vi "SaveData Loop (numpy).vi"(8 "error in":errorcluster, 10 "Message Queues out":T13, 11 "Notifiers":T1) -> (0 "error out":errorcluster)   [LabVIEW 2014]
uses:
  support/Message Queue/All Message Queues.ctl
  support/Message Queue/Message Cluster.ctl
  support/Notifiers/Notifiers.ctl
  controls/IBM OptoElectroMechanics Message Handler Loop Notifiers.ctl
  Hardware Control/HP4155C/HP4155C Notifiers.ctl
  Hardware Control/Keithley707A/Keithley 707A Notifiers.ctl
  Hardware Control/Newport ESP301/StressControl Notifiers.ctl
  Hardware Control/NGSLabspec/LabramHR Notifiers.ctl
  Hardware Control/Switches and Mirrors/SwitchesMirrors Notifiers.ctl
  Hardware Control/Camera/Camera Notifiers.ctl
  Hardware Control/Tango XYZ Stage/Tango Notifications.ctl
  Hardware Control/Autofocus/Autofocus Notifiers.ctl
  Measurements/Save Data/SaveData Notifiers.ctl
  Measurements/Instrument Sequence/Instrument Sequence Notifiers.ctl
  Measurements/Save Data/SaveData Function.ctl
  support/Message Queue/IBM OptoElectroMechanics Message Queue.lvlib
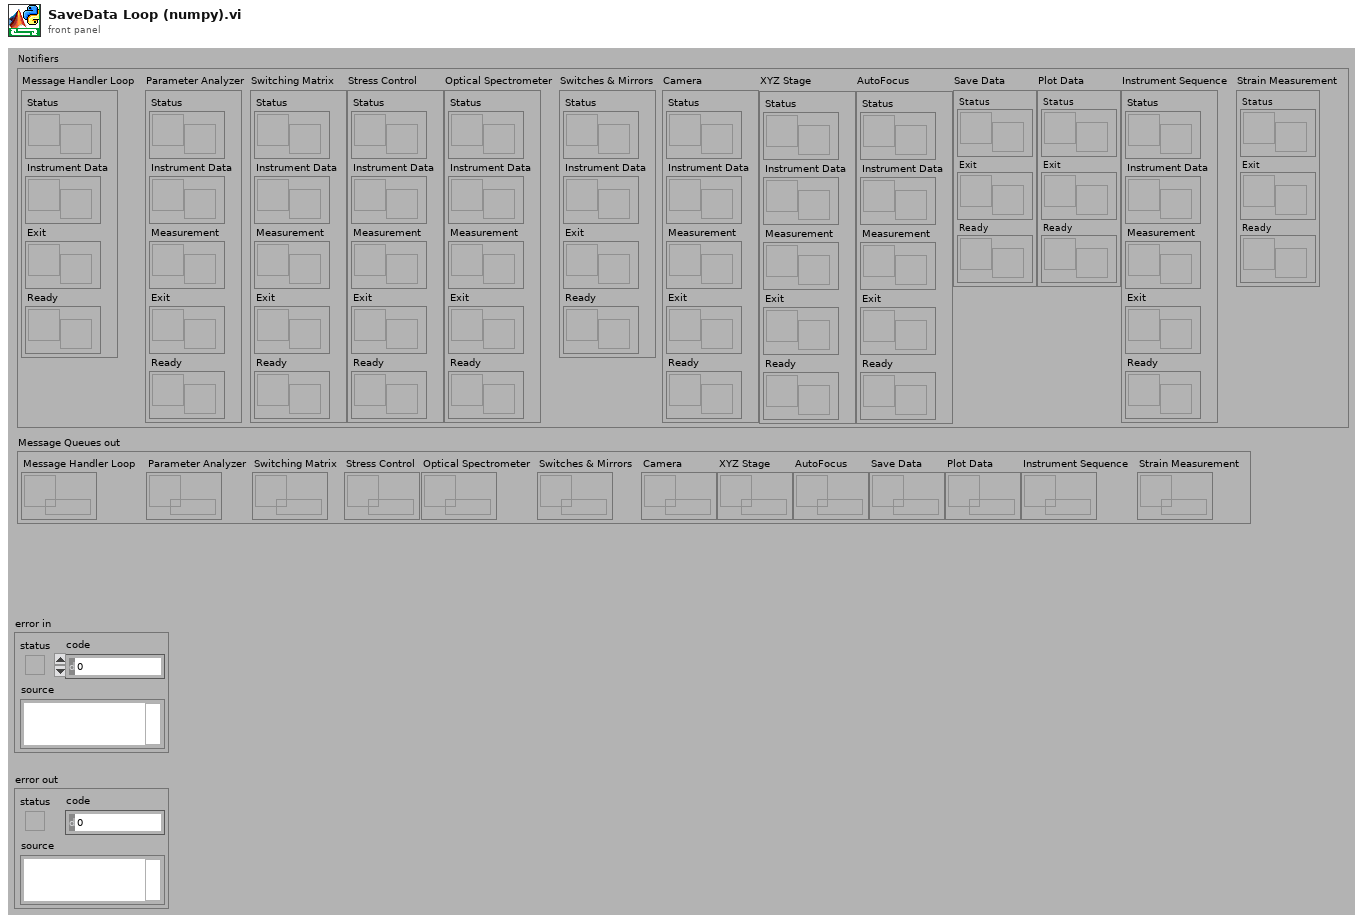
[diagram p1: front panel]
types:
  T1 = typedef "Notifiers.ctl" = cluster{"Message Handler Loop":T2, "Parameter Analyzer":T3, "Switching Matrix":T4, "Stress Control":T5, "Optical Spectrometer":T6, "Switches & Mirrors":T7, "Camera":T8, "XYZ Stage":T9, "AutoFocus":T10, "Save Data":T11, "Plot Data":T11, "Instrument Sequence":T12, "Strain Measurement":cluster{"Status":refnum<notifier>, "Exit":refnum<notifier>, "Ready":refnum<notifier>}}
  T2 = typedef "IBM OptoElectroMechanics Message Handler Loop Notifiers.ctl" = cluster{"Status":refnum<notifier>, "Instrument Data":refnum<notifier>, "Exit":refnum<notifier>, "Ready":refnum<notifier>}
  T3 = typedef "HP4155C Notifiers.ctl" = cluster{"Status":refnum<notifier>, "Instrument Data":refnum<notifier>, "Measurement":refnum<notifier>, "Exit":refnum<notifier>, "Ready":refnum<notifier>}
  T4 = typedef "Keithley 707A Notifiers.ctl" = cluster{"Status":refnum<notifier>, "Instrument Data":refnum<notifier>, "Measurement":refnum<notifier>, "Exit":refnum<notifier>, "Ready":refnum<notifier>}
  T5 = typedef "StressControl Notifiers.ctl" = cluster{"Status":refnum<notifier>, "Instrument Data":refnum<notifier>, "Measurement":refnum<notifier>, "Exit":refnum<notifier>, "Ready":refnum<notifier>}
  T6 = typedef "LabramHR Notifiers.ctl" = cluster{"Status":refnum<notifier>, "Instrument Data":refnum<notifier>, "Measurement":refnum<notifier>, "Exit":refnum<notifier>, "Ready":refnum<notifier>}
  T7 = typedef "SwitchesMirrors Notifiers.ctl" = cluster{"Status":refnum<notifier>, "Instrument Data":refnum<notifier>, "Exit":refnum<notifier>, "Ready":refnum<notifier>}
  T8 = typedef "Camera Notifiers.ctl" = cluster{"Status":refnum<notifier>, "Instrument Data":refnum<notifier>, "Measurement":refnum<notifier>, "Exit":refnum<notifier>, "Ready":refnum<notifier>}
  T9 = typedef "Tango Notifications.ctl" = cluster{"Status":refnum<notifier>, "Instrument Data":refnum<notifier>, "Measurement":refnum<notifier>, "Exit":refnum<notifier>, "Ready":refnum<notifier>}
  T10 = typedef "Autofocus Notifiers.ctl" = cluster{"Status":refnum<notifier>, "Instrument Data":refnum<notifier>, "Measurement":refnum<notifier>, "Exit":refnum<notifier>, "Ready":refnum<notifier>}
  T11 = typedef "SaveData Notifiers.ctl" = cluster{"Status":refnum<notifier>, "Exit":refnum<notifier>, "Ready":refnum<notifier>}
  T12 = typedef "Instrument Sequence Notifiers.ctl" = cluster{"Status":refnum<notifier>, "Instrument Data":refnum<notifier>, "Measurement":refnum<notifier>, "Exit":refnum<notifier>, "Ready":refnum<notifier>}
  T13 = typedef "IBM OptoElectroMechanics Message Queue.lvlib/All Message Queues.ctl" = cluster{"Message Handler Loop":refnum<queue>, "Parameter Analyzer":refnum<queue>, "Switching Matrix":refnum<queue>, "Stress Control":refnum<queue>, "Optical Spectrometer":refnum<queue>, "Switches & Mirrors":refnum<queue>, "Camera":refnum<queue>, "XYZ Stage":refnum<queue>, "AutoFocus":refnum<queue>, "Save Data":refnum<queue>, "Plot Data":refnum<queue>, "Instrument Sequence":refnum<queue>, "Strain Measurement":refnum<queue>}
  T14 = typedef "SaveData Function.ctl" = enum16{"Start Python Session", "Set Data Structures to Default", "Append Stress Data", "Append Electrical Measurement", "Append Optical Spectrum", "Append Stress Measurement Step", "Append Instrument Sequence Step", "Set Instrument Configuration", "Set Stress Data", "Set Electrical Measurement", "Set Optical Spectum", "Save Electrical Measurement", "Save Optical Spectrum", "Save Instrument Sequence", "Save Stress Measurement", "Pickle2Workspace", "Explore Variable Space", "Close"}
  T15 = typedef "SaveData Data.ctl" = cluster{"Configuration":T16, "Initialization":T21}
  T16 = typedef "SaveData Config.ctl" = cluster{"Workspace Info":T17, "Instrument Configuration":T18, "Stress Motor Position":dbl, "Electrical Measurement":cluster{"Sequence":dbl[], "V1":dbl[], "V2":dbl[], "V3":dbl[], "V4":dbl[], "I1":dbl[], "I2":dbl[], "I3":dbl[], "I4":dbl[]}, "Optical Spectrum":T20}
  T17 = typedef "SaveData Workspace Info.ctl" = cluster{"Device Name":string, "Device Info":string, "Path":path}
  T18 = typedef "SaveData Instrument Configuration.ctl" = cluster{"Instrument":T19, "Configuration":string}
  T19 = typedef "Instrument List.ctl" = enum32{"Unknown Instrument", "Switching Matrix", "Parameter Analyzer", "Optical Spectrometer"}
  T20 = typedef "Spectral Data.ctl" = cluster{"Intensity":dbl[], "Wavelength":dbl[], "Energy":dbl[], "Raman Shift":dbl[], "Detector Temperature":dbl}
  T21 = typedef "SaveData Initialization.ctl" = cluster{"Start Python Session":bool, "Set Datastructures to Default":bool}
  T22 = cluster{"Sequence":dbl[], "V1":dbl[], "V2":dbl[], "V3":dbl[], "V4":dbl[], "I1":dbl[], "I2":dbl[], "I3":dbl[], "I4":dbl[]}
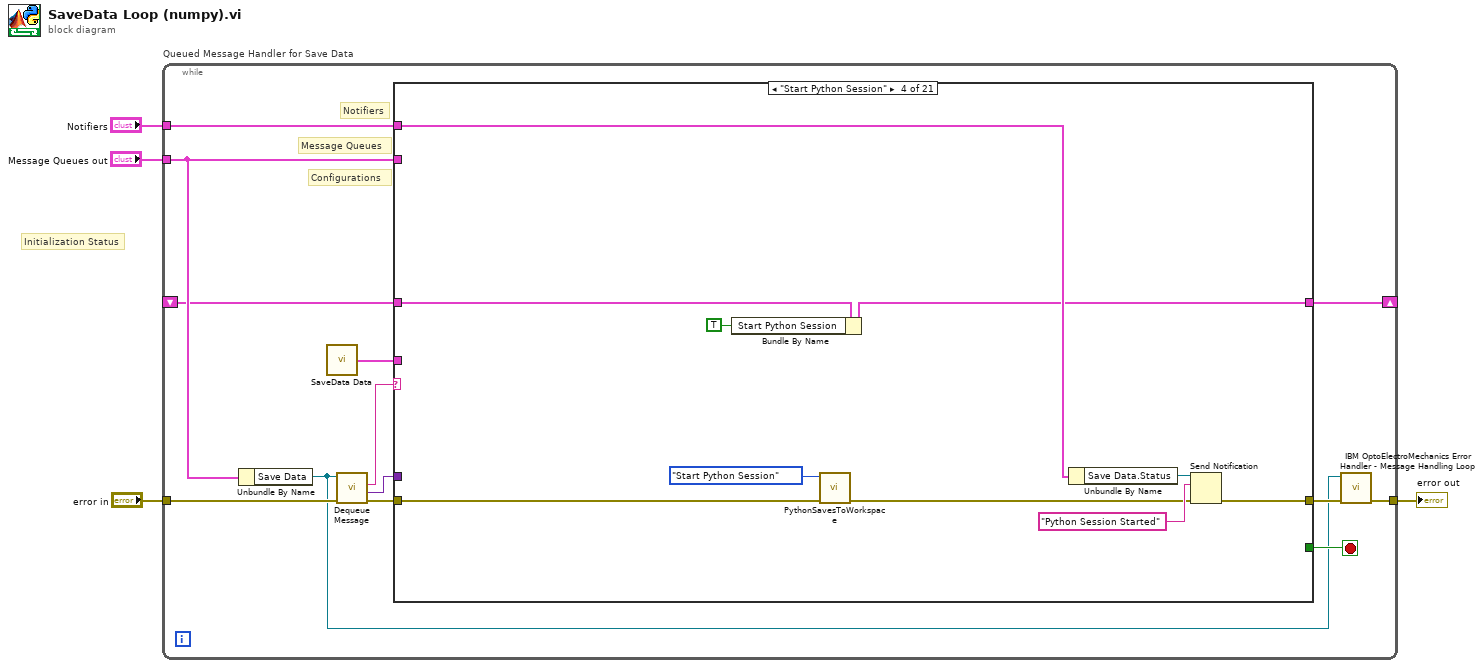
[diagram p0: block diagram]
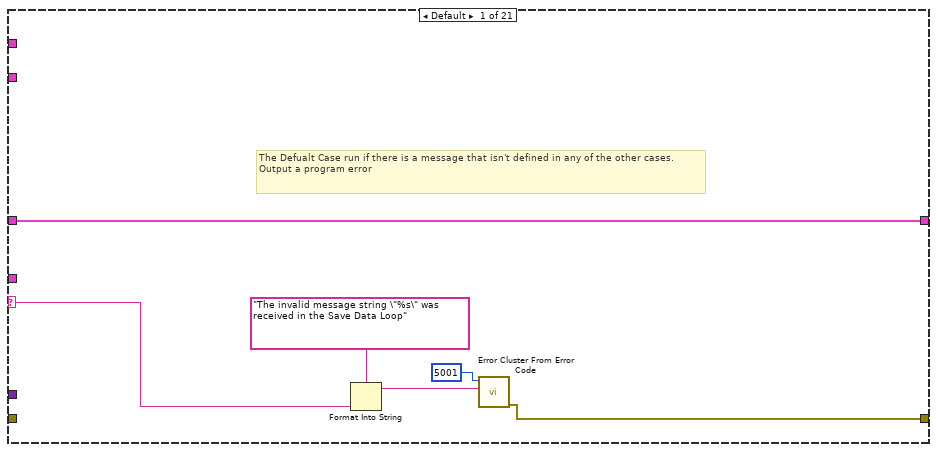
[diagram p2: hidden frame]
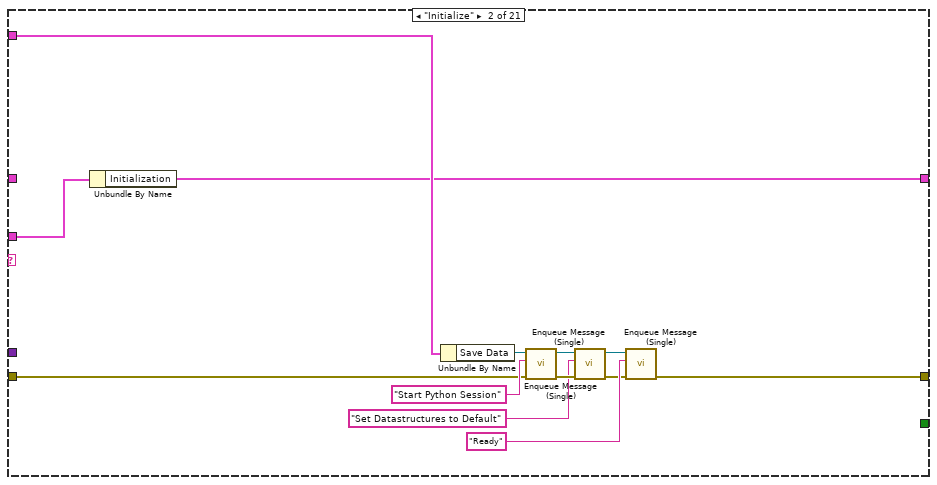
[diagram p3: hidden frame]
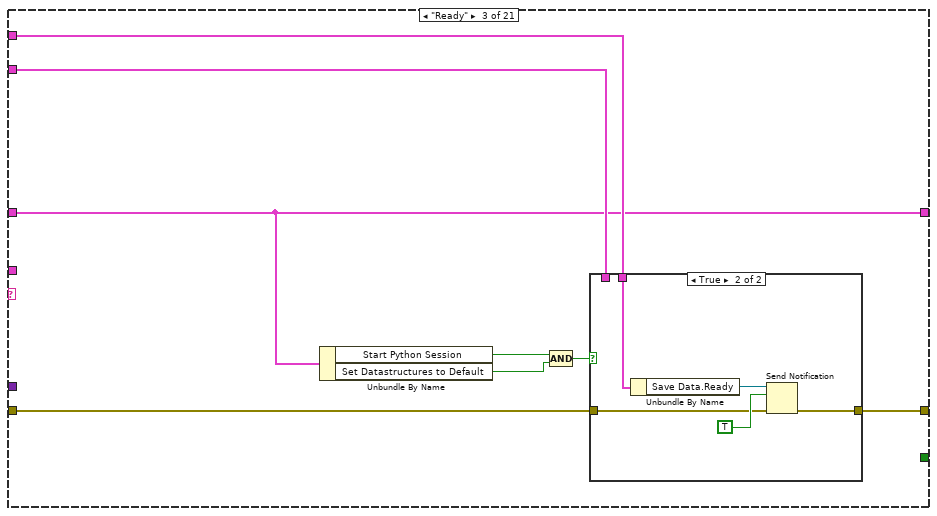
[diagram p4: hidden frame]
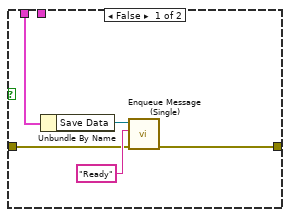
[diagram p5: hidden frame]
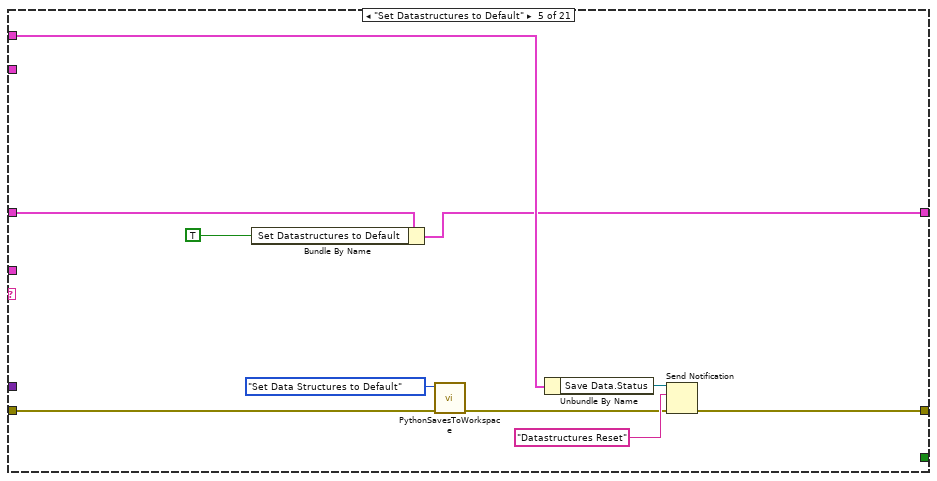
[diagram p6: hidden frame]
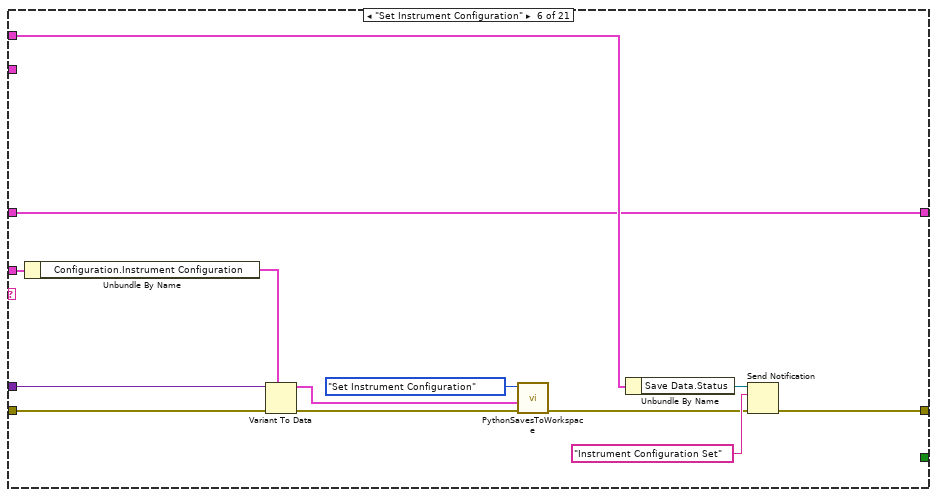
[diagram p7: hidden frame]
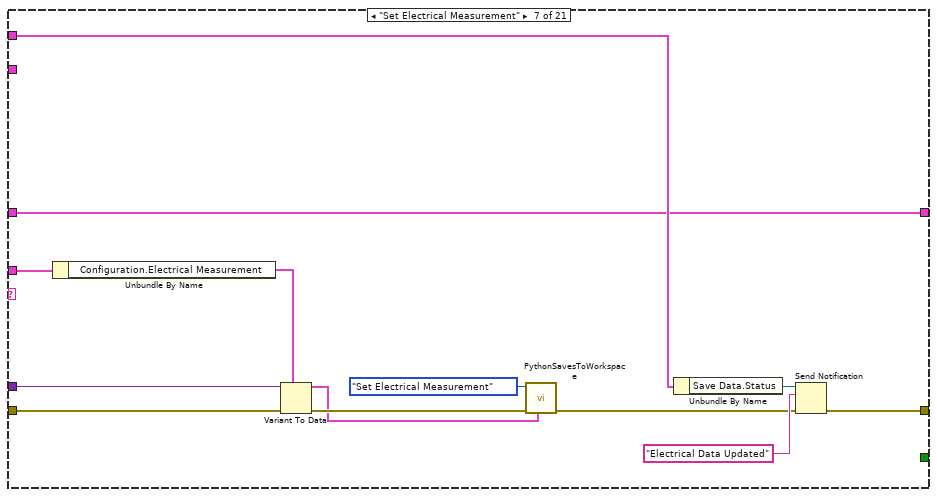
[diagram p8: hidden frame]
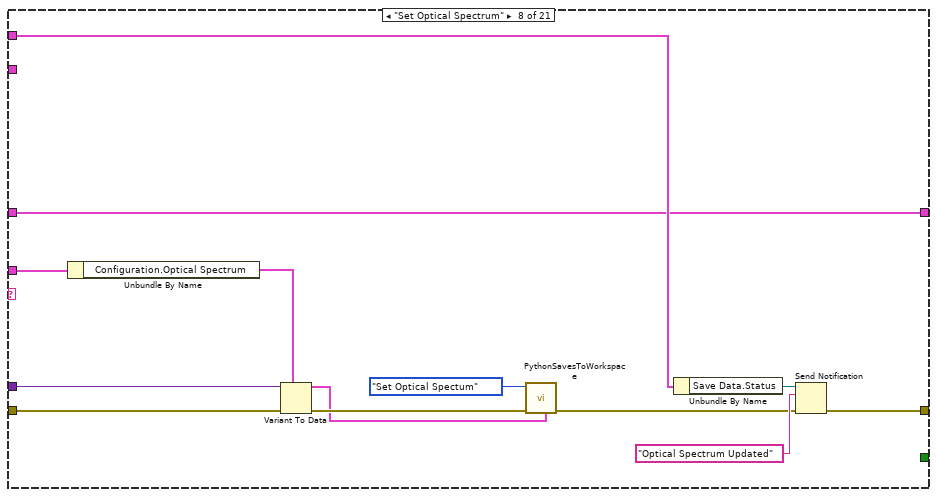
[diagram p9: hidden frame]
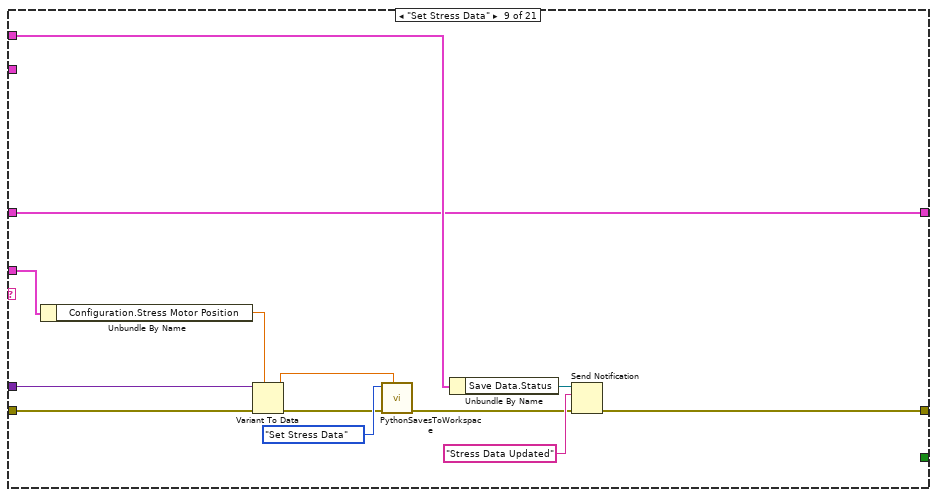
[diagram p10: hidden frame]
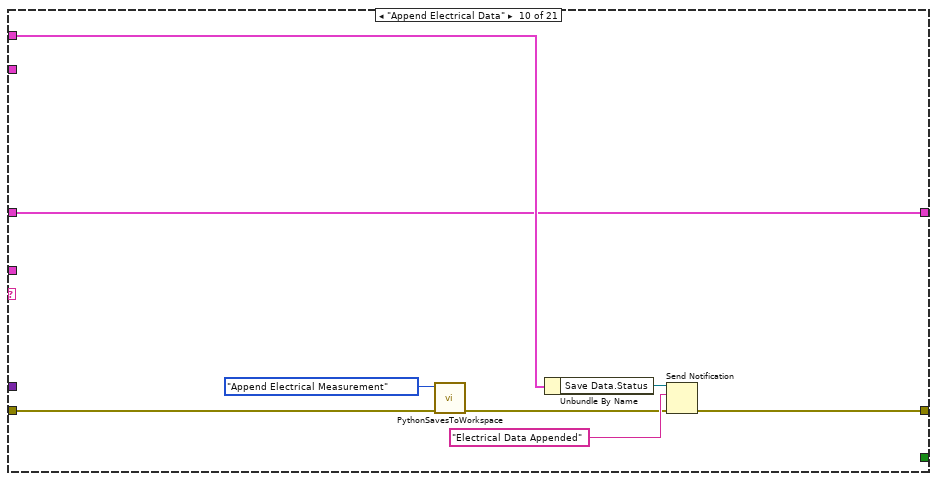
[diagram p11: hidden frame]
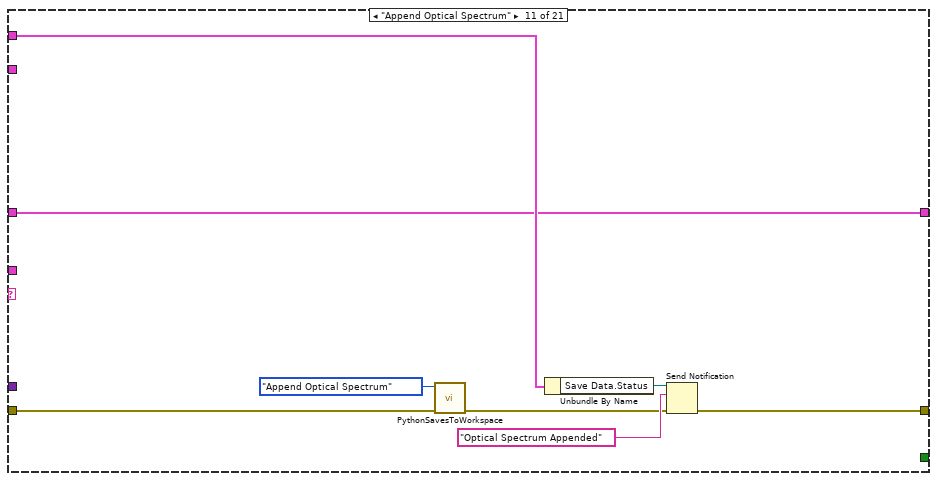
[diagram p12: hidden frame]
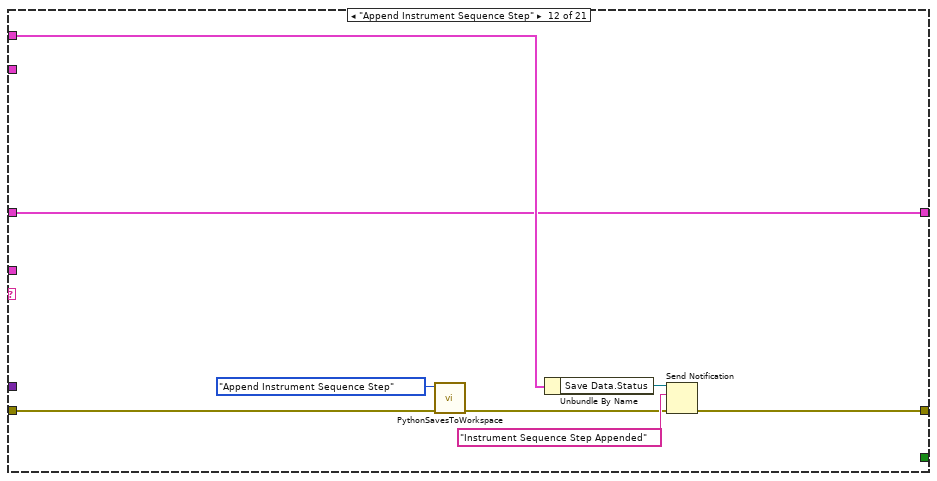
[diagram p13: hidden frame]
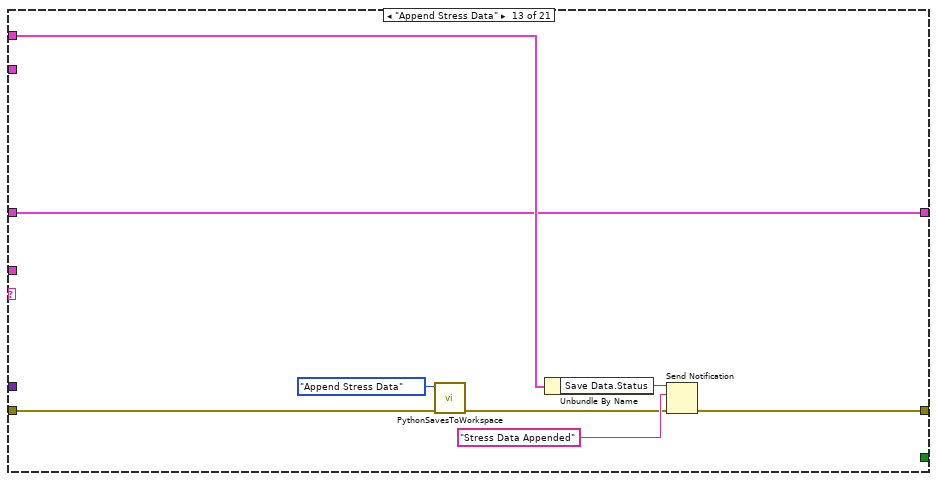
[diagram p14: hidden frame]
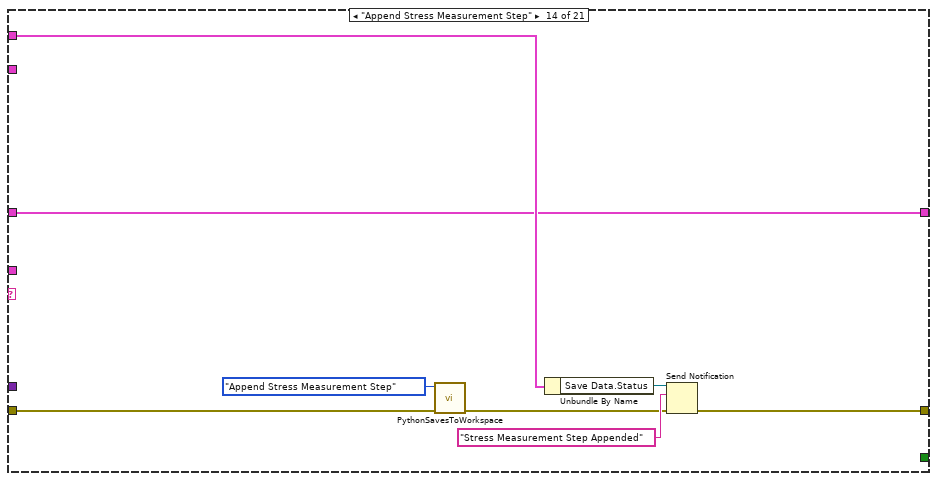
[diagram p15: hidden frame]
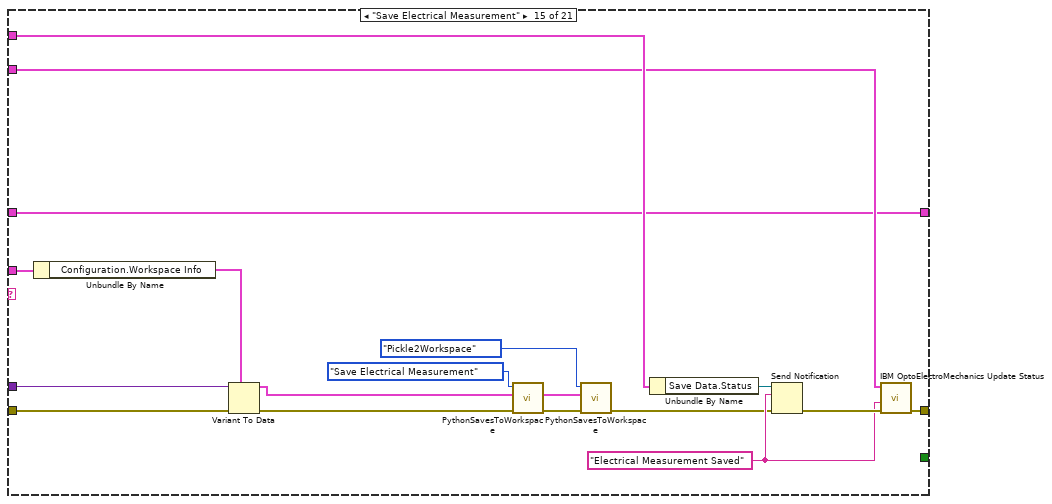
[diagram p16: hidden frame]
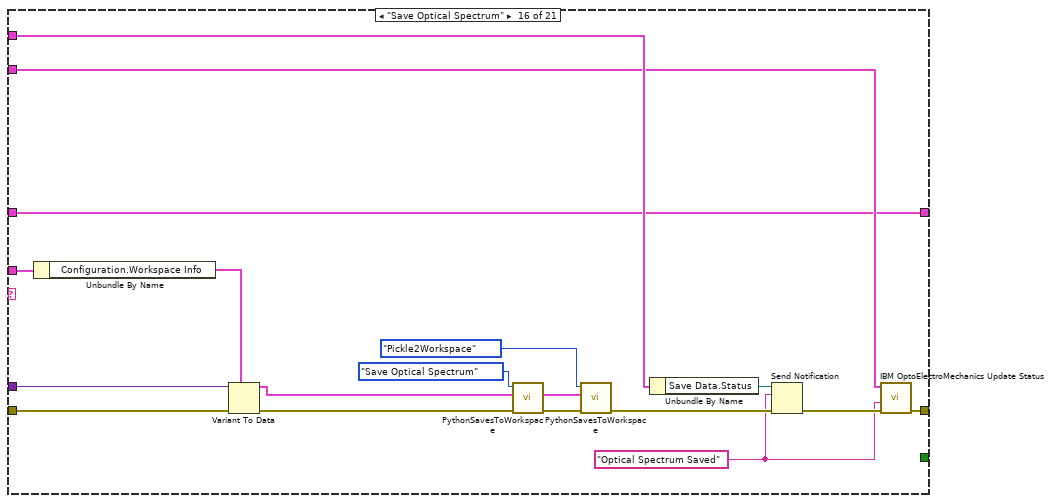
[diagram p17: hidden frame]
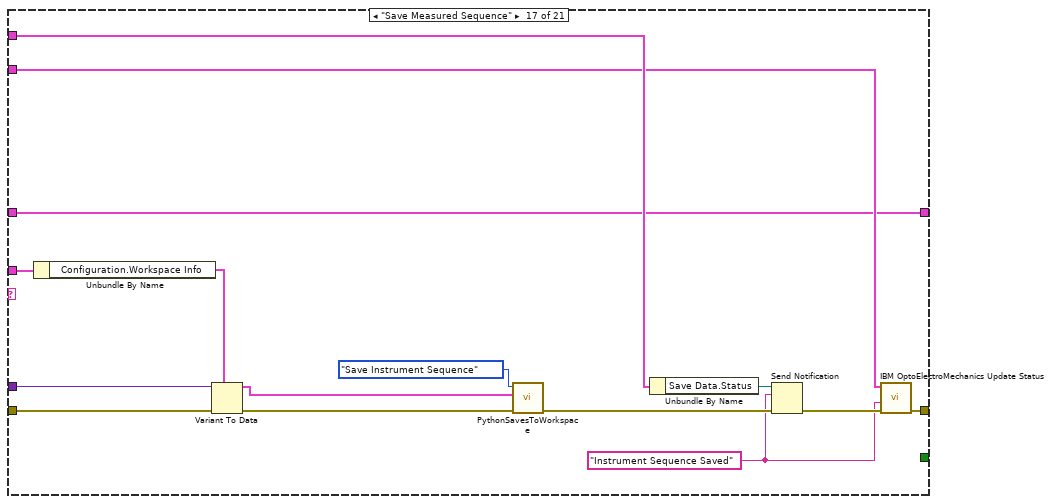
[diagram p18: hidden frame]
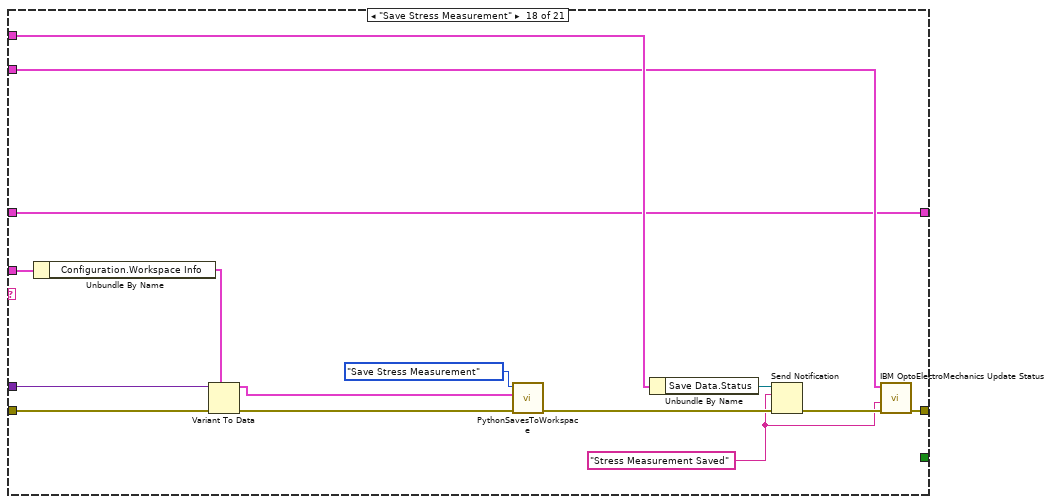
[diagram p19: hidden frame]
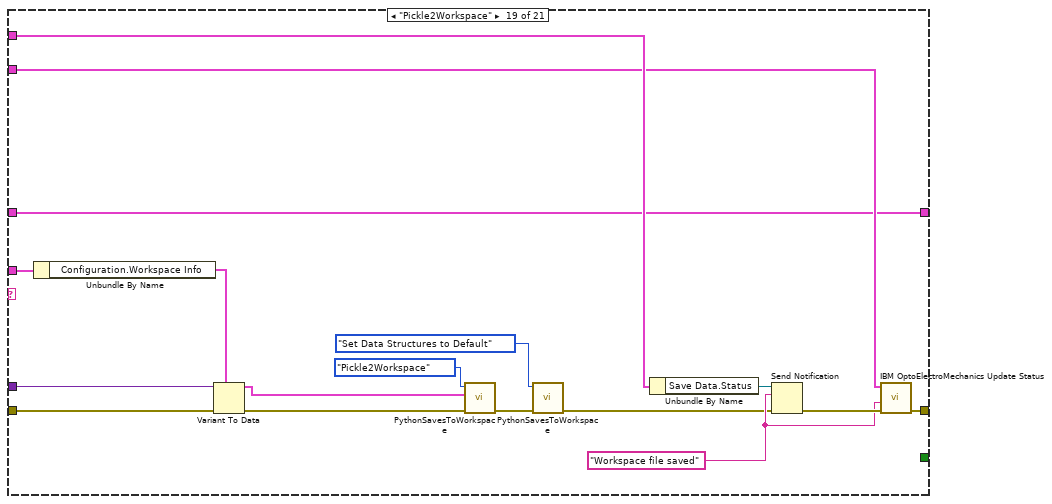
[diagram p20: hidden frame]
diagram:
  # "Initialization Status"
  n1 = while "Queued Message Handler for Save Data" {
    tunnel: "error in" -> [w17]
    tunnel: [w9] -> w1
    tunnel: "Message Queues out" -> [w13]
    tunnel: "Notifiers" -> [w12]
    shift-right: [w6] -> _
    shift-left: _ -> [w5]
    stop <- w11 stop-if-true
    # "Configurations"
    # "Notifiers"
    # "Message Queues"
    n2 = Unbundle By Name(w13) -> ("Save Data"=w8:refnum<queue>)
    n3 = call "SaveData Data.vi"() -> ("SavaData Data"=w7:T15)
    n4 = call "Dequeue Message.vi"("error in (no error)"=w17, "Message Queue"=w8) -> ("error out"=w16:errorcluster, "Message Data"=w14:variant, "Message"=w15:string)  [unwired: 7 out]
    n5 = case shown="\"Start Python Session\"" w15 {
      selector: w15 -> [w20 _ _ _ _ _ _ _ _ _ _ _ _ _ _ _ _ _ _ _ _]
      tunnel: w16 -> [_ w33 w44 w62 w72 w87 w100 w113 w126 w133 w141 w149 w157 w165 w183 w200 w215 w230 w247 w256 w269]
      tunnel: [w19 w26 w42 w57 w67 w78 w90 w104 w116 w128 w136 w144 w152 w160 w178 w195 w210 w225 w242 w251 w264] -> w10
      tunnel: w14 -> [_ _ _ _ _ w86 w99 w112 w125 _ _ _ _ _ w182 w199 w214 w229 w246 w249 _]
      tunnel: w13 -> [_ w36 w43 _ _ _ _ _ _ _ _ _ _ _ w179 w196 w211 w226 w243 w257 w275]
      tunnel: w12 -> [_ _ w41 w59 w69 w85 w98 w111 w124 w130 w138 w146 w154 w162 w181 w198 w213 w228 w245 _ w270]
      tunnel: [_ _ _ _ _ _ _ _ _ _ _ _ _ _ _ _ _ _ _ _ TRUE ("Priority Message? (F)")] -> w11
      tunnel: w7 -> [_ w25 _ _ _ w77 w89 w103 w115 _ _ _ _ _ w172 w190 w203 w218 w236 _ w266]
      tunnel: [w18 w24 w37 w56 w65 w75 w88 w102 w114 w127 w135 w143 w151 w159 w171 w189 w202 w217 w235 w248 w265] -> w6
      tunnel: w5 -> [w18 _ w37 w55 w66 w75 w88 w102 w114 w127 w135 w143 w151 w159 w171 w189 w202 w217 w235 w248 _]
      frame Default {
        # "The Defualt Case run if there is a message that isn't defined in any of the other cases.\nOutput a program error"
        n6 = Format Into String(format string="The invalid message string \"%s\" was  received in the Save Data Loop", w20) -> (resulting string=w22:string)  [unwired: 2 in, 1 out]
        n7 = call <vilib>:"Error Cluster From Error Code.vi"("error message (\"\")"=w22, "error code (0)"=5001) -> ("error out"=w19:errorcluster)  [unwired: 2 in, 5 out]
      }
      frame "Initialize" {
        n8 = Unbundle By Name(w25) -> ("Initialization"=w24:T21)
        n9 = Unbundle By Name(w36) -> ("Save Data"=w34:refnum<queue>)
        n10 = call "Enqueue Message (Single).vi"("error in (no error)"=w33, "Message"="Start Python Session", "Message Queue"=w34) -> ("error out"=w32:errorcluster, "dup Message Queue"=w31:refnum<queue>)  [unwired: 1 in, 6 out]
        n11 = call "Enqueue Message (Single).vi"("error in (no error)"=w32, "Message"="Set Datastructures to Default", "Message Queue"=w31) -> ("error out"=w27:errorcluster, "dup Message Queue"=w29:refnum<queue>)  [unwired: 1 in, 6 out]
        n12 = call "Enqueue Message (Single).vi"("error in (no error)"=w27, "Message"="Ready", "Message Queue"=w29) -> ("error out"=w26:errorcluster)  [unwired: 1 in, 7 out]
      }
      frame "Ready" {
        n13 = Unbundle By Name(w37) -> ("Start Python Session"=w40:bool, "Set Datastructures to Default"=w38:bool)
        n14 = Compound Arithmetic op=AND(w40, w38) -> (w39:bool)
        n15 = case shown="True" w39 {
          tunnel: [w47 w52] -> w42
          tunnel: w44 -> [w46 w51]
          tunnel: w43 -> [w45 _]
          tunnel: w41 -> [_ w50]
          frame False {
            n16 = Unbundle By Name(w45) -> ("Save Data"=w49:refnum<queue>)
            n17 = call "Enqueue Message (Single).vi"("error in (no error)"=w46, "Message"="Ready", "Message Queue"=w49) -> ("error out"=w47:errorcluster)  [unwired: 1 in, 7 out]
          }
          frame True {
            n18 = Unbundle By Name(w50) -> ("Save Data.Ready"=w53:refnum<notifier>)
            n19 = Send Notification(notification=TRUE, notifier=w53, error in (no error)=w51) -> (error out=w52:errorcluster)  [unwired: 1 out]
          }
        }
      }
      frame "Start Python Session" {
        n20 = Bundle By Name(cluster=w55, "Start Python Session"=TRUE ("Initialization.Open VI reference")) -> (w56:T21)
        n21 = call "PythonSavesToWorkspace.vi"("error in (no error)"=w62, "Function"=SaveData_Function."Start Python Session") -> ("error out"=w58:errorcluster)  [unwired: 5 in, 4 out]
        n22 = Unbundle By Name(w59) -> ("Save Data.Status"=w60:refnum<notifier>)
        n23 = Send Notification(notification="Python Session Started", notifier=w60, error in (no error)=w58) -> (error out=w57:errorcluster)  [unwired: 1 out]
      }
      frame "Set Datastructures to Default" {
        n24 = Bundle By Name(cluster=w66, "Set Datastructures to Default"=TRUE ("Initialization.Open VI reference")) -> (w65:T21)
        n25 = call "PythonSavesToWorkspace.vi"("error in (no error)"=w72, "Function"=SaveData_Function."Set Data Structures to Default") -> ("error out"=w68:errorcluster)  [unwired: 5 in, 4 out]
        n26 = Unbundle By Name(w69) -> ("Save Data.Status"=w70:refnum<notifier>)
        n27 = Send Notification(notification="Datastructures Reset", notifier=w70, error in (no error)=w68) -> (error out=w67:errorcluster)  [unwired: 1 out]
      }
      frame "Set Instrument Configuration" {
        n28 = Unbundle By Name(w77) -> ("Configuration.Instrument Configuration"=w84:T18)
        n29 = Variant To Data(error in=w87, type=w84, Variant=w86) -> (data=w76:T18, error out=w79:errorcluster)
        n30 = call "PythonSavesToWorkspace.vi"("error in (no error)"=w79, "Instrument Configuration"=w76, "Function"=SaveData_Function."Set Instrument Configuration") -> ("error out"=w80:errorcluster)  [unwired: 4 in, 4 out]
        n31 = Unbundle By Name(w85) -> ("Save Data.Status"=w82:refnum<notifier>)
        n32 = Send Notification(notification="Instrument Configuration Set", notifier=w82, error in (no error)=w80) -> (error out=w78:errorcluster)  [unwired: 1 out]
      }
      frame "Set Electrical Measurement" {
        n33 = Unbundle By Name(w89) -> ("Configuration.Electrical Measurement"=w97:T22)
        n34 = Variant To Data(error in=w100, type=w97, Variant=w99) -> (data=w91:T22, error out=w92:errorcluster)
        n35 = call "PythonSavesToWorkspace.vi"("Electrical Measurement"=w91, "error in (no error)"=w92, "Function"=SaveData_Function."Set Electrical Measurement") -> ("error out"=w93:errorcluster)  [unwired: 4 in, 4 out]
        n36 = Unbundle By Name(w98) -> ("Save Data.Status"=w95:refnum<notifier>)
        n37 = Send Notification(notification="Electrical Data Updated", notifier=w95, error in (no error)=w93) -> (error out=w90:errorcluster)  [unwired: 1 out]
      }
      frame "Set Optical Spectrum" {
        n38 = Unbundle By Name(w103) -> ("Configuration.Optical Spectrum"=w110:T20)
        n39 = Variant To Data(error in=w113, type=w110, Variant=w112) -> (data=w101:T20, error out=w105:errorcluster)
        n40 = call "PythonSavesToWorkspace.vi"("Optical Spectrum"=w101, "error in (no error)"=w105, "Function"=SaveData_Function."Set Optical Spectum") -> ("error out"=w106:errorcluster)  [unwired: 4 in, 4 out]
        n41 = Unbundle By Name(w111) -> ("Save Data.Status"=w108:refnum<notifier>)
        n42 = Send Notification(notification="Optical Spectrum Updated", notifier=w108, error in (no error)=w106) -> (error out=w104:errorcluster)  [unwired: 1 out]
      }
      frame "Set Stress Data" {
        n43 = Unbundle By Name(w115) -> ("Configuration.Stress Motor Position"=w123:dbl)
        n44 = Variant To Data(error in=w126, type=w123, Variant=w125) -> (data=w117:dbl, error out=w118:errorcluster)
        n45 = call "PythonSavesToWorkspace.vi"("Stress Motor Position"=w117, "error in (no error)"=w118, "Function"=SaveData_Function."Set Stress Data") -> ("error out"=w119:errorcluster)  [unwired: 4 in, 4 out]
        n46 = Unbundle By Name(w124) -> ("Save Data.Status"=w121:refnum<notifier>)
        n47 = Send Notification(notification="Stress Data Updated", notifier=w121, error in (no error)=w119) -> (error out=w116:errorcluster)  [unwired: 1 out]
      }
      frame "Append Electrical Data" {
        n48 = call "PythonSavesToWorkspace.vi"("error in (no error)"=w133, "Function"=SaveData_Function."Append Electrical Measurement") -> ("error out"=w129:errorcluster)  [unwired: 5 in, 4 out]
        n49 = Unbundle By Name(w130) -> ("Save Data.Status"=w131:refnum<notifier>)
        n50 = Send Notification(notification="Electrical Data Appended", notifier=w131, error in (no error)=w129) -> (error out=w128:errorcluster)  [unwired: 1 out]
      }
      frame "Append Optical Spectrum" {
        n51 = call "PythonSavesToWorkspace.vi"("error in (no error)"=w141, "Function"=SaveData_Function."Append Optical Spectrum") -> ("error out"=w137:errorcluster)  [unwired: 5 in, 4 out]
        n52 = Unbundle By Name(w138) -> ("Save Data.Status"=w139:refnum<notifier>)
        n53 = Send Notification(notification="Optical Spectrum Appended", notifier=w139, error in (no error)=w137) -> (error out=w136:errorcluster)  [unwired: 1 out]
      }
      frame "Append Instrument Sequence Step" {
        n54 = call "PythonSavesToWorkspace.vi"("error in (no error)"=w149, "Function"=SaveData_Function."Append Instrument Sequence Step") -> ("error out"=w145:errorcluster)  [unwired: 5 in, 4 out]
        n55 = Unbundle By Name(w146) -> ("Save Data.Status"=w147:refnum<notifier>)
        n56 = Send Notification(notification="Instrument Sequence Step Appended", notifier=w147, error in (no error)=w145) -> (error out=w144:errorcluster)  [unwired: 1 out]
      }
      frame "Append Stress Data" {
        n57 = call "PythonSavesToWorkspace.vi"("error in (no error)"=w157, "Function"=SaveData_Function."Append Stress Data") -> ("error out"=w153:errorcluster)  [unwired: 5 in, 4 out]
        n58 = Unbundle By Name(w154) -> ("Save Data.Status"=w155:refnum<notifier>)
        n59 = Send Notification(notification="Stress Data Appended", notifier=w155, error in (no error)=w153) -> (error out=w152:errorcluster)  [unwired: 1 out]
      }
      frame "Append Stress Measurement Step" {
        n60 = call "PythonSavesToWorkspace.vi"("error in (no error)"=w165, "Function"=SaveData_Function."Append Stress Measurement Step") -> ("error out"=w161:errorcluster)  [unwired: 5 in, 4 out]
        n61 = Unbundle By Name(w162) -> ("Save Data.Status"=w163:refnum<notifier>)
        n62 = Send Notification(notification="Stress Measurement Step Appended", notifier=w163, error in (no error)=w161) -> (error out=w160:errorcluster)  [unwired: 1 out]
      }
      frame "Save Electrical Measurement" {
        w173 = "Electrical Measurement Saved"
        n63 = Unbundle By Name(w172) -> ("Configuration.Workspace Info"=w176:T17)
        n64 = Variant To Data(error in=w183, type=w176, Variant=w182) -> (data=w167:T17, error out=w174:errorcluster)
        n65 = call "PythonSavesToWorkspace.vi"("error in (no error)"=w174, "Workspace Info"=w167, "Function"=SaveData_Function."Save Electrical Measurement") -> ("error out"=w169:errorcluster)  [unwired: 4 in, 4 out]
        n66 = call "PythonSavesToWorkspace.vi"("error in (no error)"=w169, "Workspace Info"=w167, "Function"=SaveData_Function."Pickle2Workspace") -> ("error out"=w168:errorcluster)  [unwired: 4 in, 4 out]
        n67 = Unbundle By Name(w181) -> ("Save Data.Status"=w177:refnum<notifier>)
        n68 = Send Notification(notification=w173, notifier=w177, error in (no error)=w168) -> (error out=w180:errorcluster)  [unwired: 1 out]
        n69 = call "IBM OptoElectroMechanics Update Status.vi"("error in"=w180, "String"=w173, "Message Queues out"=w179) -> ("error out"=w178:errorcluster)  [unwired: 8 out]
      }
      frame "Save Optical Spectrum" {
        w184 = "Optical Spectrum Saved"
        n70 = Unbundle By Name(w190) -> ("Configuration.Workspace Info"=w193:T17)
        n71 = Variant To Data(error in=w200, type=w193, Variant=w199) -> (data=w185:T17, error out=w191:errorcluster)
        n72 = call "PythonSavesToWorkspace.vi"("error in (no error)"=w191, "Workspace Info"=w185, "Function"=SaveData_Function."Save Optical Spectrum") -> ("error out"=w187:errorcluster)  [unwired: 4 in, 4 out]
        n73 = call "PythonSavesToWorkspace.vi"("error in (no error)"=w187, "Workspace Info"=w185, "Function"=SaveData_Function."Pickle2Workspace") -> ("error out"=w186:errorcluster)  [unwired: 4 in, 4 out]
        n74 = Unbundle By Name(w198) -> ("Save Data.Status"=w194:refnum<notifier>)
        n75 = Send Notification(notification=w184, notifier=w194, error in (no error)=w186) -> (error out=w197:errorcluster)  [unwired: 1 out]
        n76 = call "IBM OptoElectroMechanics Update Status.vi"("error in"=w197, "String"=w184, "Message Queues out"=w196) -> ("error out"=w195:errorcluster)  [unwired: 8 out]
      }
      frame "Save Measured Sequence" {
        w204 = "Instrument Sequence Saved"
        n77 = Unbundle By Name(w203) -> ("Configuration.Workspace Info"=w208:T17)
        n78 = Variant To Data(error in=w215, type=w208, Variant=w214) -> (data=w201:T17, error out=w205:errorcluster)
        n79 = call "PythonSavesToWorkspace.vi"("error in (no error)"=w205, "Workspace Info"=w201, "Function"=SaveData_Function."Save Instrument Sequence") -> ("error out"=w206:errorcluster)  [unwired: 4 in, 4 out]
        n80 = Unbundle By Name(w213) -> ("Save Data.Status"=w209:refnum<notifier>)
        n81 = Send Notification(notification=w204, notifier=w209, error in (no error)=w206) -> (error out=w212:errorcluster)  [unwired: 1 out]
        n82 = call "IBM OptoElectroMechanics Update Status.vi"("error in"=w212, "String"=w204, "Message Queues out"=w211) -> ("error out"=w210:errorcluster)  [unwired: 8 out]
      }
      frame "Save Stress Measurement" {
        w219 = "Stress Measurement Saved"
        n83 = Unbundle By Name(w218) -> ("Configuration.Workspace Info"=w223:T17)
        n84 = Variant To Data(error in=w230, type=w223, Variant=w229) -> (data=w216:T17, error out=w220:errorcluster)
        n85 = call "PythonSavesToWorkspace.vi"("error in (no error)"=w220, "Workspace Info"=w216, "Function"=SaveData_Function."Save Stress Measurement") -> ("error out"=w221:errorcluster)  [unwired: 4 in, 4 out]
        n86 = Unbundle By Name(w228) -> ("Save Data.Status"=w224:refnum<notifier>)
        n87 = Send Notification(notification=w219, notifier=w224, error in (no error)=w221) -> (error out=w227:errorcluster)  [unwired: 1 out]
        n88 = call "IBM OptoElectroMechanics Update Status.vi"("error in"=w227, "String"=w219, "Message Queues out"=w226) -> ("error out"=w225:errorcluster)  [unwired: 8 out]
      }
      frame "Pickle2Workspace" {
        w237 = "Workspace file saved"
        n89 = Unbundle By Name(w236) -> ("Configuration.Workspace Info"=w240:T17)
        n90 = Variant To Data(error in=w247, type=w240, Variant=w246) -> (data=w231:T17, error out=w238:errorcluster)
        n91 = call "PythonSavesToWorkspace.vi"("error in (no error)"=w238, "Workspace Info"=w231, "Function"=SaveData_Function."Pickle2Workspace") -> ("error out"=w233:errorcluster)  [unwired: 4 in, 4 out]
        n92 = call "PythonSavesToWorkspace.vi"("error in (no error)"=w233, "Function"=SaveData_Function."Set Data Structures to Default") -> ("error out"=w232:errorcluster)  [unwired: 5 in, 4 out]
        n93 = Unbundle By Name(w245) -> ("Save Data.Status"=w241:refnum<notifier>)
        n94 = Send Notification(notification=w237, notifier=w241, error in (no error)=w232) -> (error out=w244:errorcluster)  [unwired: 1 out]
        n95 = call "IBM OptoElectroMechanics Update Status.vi"("error in"=w244, "String"=w237, "Message Queues out"=w243) -> ("error out"=w242:errorcluster)  [unwired: 8 out]
      }
      frame "Error" {
        # "Clear Errors to avoid getting stuck \nin repeating this case"
        # "Add here Cases that are handled \nalready by the Message Handler Loop"
        n96 = Variant To Data(error in=w256, type=errorcluster {"status"=FALSE, "code"=0, "source"=""} ("error out"), Variant=w249) -> (data=w255:errorcluster, error out=w254:errorcluster)
        n97 = Merge Errors(w255, w254) -> (w253:errorcluster)
        n98 = Unbundle By Name(w257) -> ("Message Handler Loop"=w259:refnum<queue>)
        n99 = Unbundle By Name(w253) -> ("code"=w250:i32)
        n100 = case shown="Default" w250 {
          tunnel: w259 -> [w263]
          tunnel: w253 -> [w261]
          tunnel: [w260] -> w252
          frame Default {
            n101 = call "Enqueue Message (Single).vi"("Message Data"=w261, "Message"="Error", "Message Queue"=w263) -> ("error out"=w260:errorcluster)  [unwired: 1 in, 7 out]
          }
        }
        n102 = call <vilib>:"Clear Errors.vi"("error in (no error)"=w252) -> ("error out"=w251:errorcluster)  [unwired: 1 in, 5 out]
      }
      frame "Exit" {
        # "Stop the VI"
        n103 = Unbundle By Name(w266) -> ("Initialization"=w265:T21)
        n104 = call "PythonSavesToWorkspace.vi"("error in (no error)"=w269, "Function"=SaveData_Function."Close") -> ("error out"=w268:errorcluster)  [unwired: 5 in, 4 out]
        n105 = Unbundle By Name(w275) -> ("Save Data"=w276:refnum<queue>)
        n106 = Release Queue(queue=w276, error in (no error)=w268) -> (error out=w274:errorcluster)  [unwired: 3 out]
        n107 = Unbundle By Name(w270) -> ("Save Data.Exit"=w273:refnum<notifier>)
        n108 = Send Notification(notification=FALSE ("Priority Message? (F)"), notifier=w273, error in (no error)=w274) -> (error out=w264:errorcluster)  [unwired: 1 out]
      }
    }
    n109 = call "IBM OptoElectroMechanics Error Handler - Message Handling Loop.vi"("error in (no error)"=w10, "Message Queue"=w8) -> ("dup error in"=w9:errorcluster)  [unwired: 9 out]
  }
  "error out" <- w1
